vi "Configure Instrument.vi"(8 "error in (no error)":errorcluster, 11 "VNA":refnum<class "VNA.lvclass">) -> (0 "error out":errorcluster, 3 "VNA out":refnum<class "VNA.lvclass">)   [LabVIEW 2019, in "VNA.lvclass"]
uses:
  VNA.lvclass
  <userlib>/LevyLab/Instrument Framework/Instrument Types/VNA/Instrument.VNA.lvclass
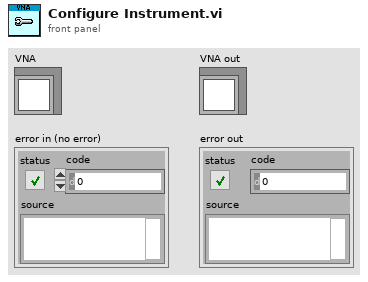
[diagram p1: front panel]
types:
  T1 = typedef "VNA.lvclass/VNA.Configuration--Cluster.ctl" = cluster{"Power":dbl, "Measurement":dbl, "Format":dbl, "Start Freq":dbl, "Stop Freq":dbl, "Num Points":dbl, "Avg Factor":dbl, "Avg?":bool, "Path":path}
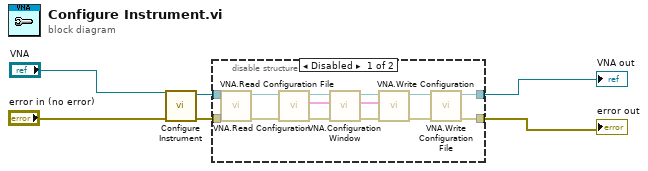
[diagram p0: block diagram]
diagram:
  n1 = call-parent "Configure Instrument.vi"("error in (no error)"="error in (no error)", "Instrument in"="VNA") -> ("error out"=w1:errorcluster, "Instrument out"=w3:refnum<class "VNA.lvclass">)  [unwired: 8 in]
  n2 = disable-structure shown="Disabled" {
    disable-tunnel: [w20 w21] -> w5
    disable-tunnel: [w19 w22] -> w4
    disable-tunnel: w3 -> [w18 w22]
    disable-tunnel: w1 -> [w17 w21]
    frame Disabled {
      n3 = call "VNA.Read Configuration File.vi"("error in (no error)"=w17, "VNA"=w18) -> ("error out"=w16:errorcluster, "VNA out"=w15:refnum<class "VNA.lvclass">)  [unwired: 8 in]
      n4 = call "VNA.Read Configuration.vi"("error in (no error)"=w16, "VNA"=w15) -> ("error out"=w13:errorcluster, "Configuration"=w8:T1, "VNA out"=w14:refnum<class "VNA.lvclass">)  [unwired: 7 in]
      n5 = call "VNA.Configuration Window.vi"("error in (no error)"=w13, "Ex Configuration"=w8, "VNA"=w14) -> ("error out"=w12:errorcluster, "output cluster"=w7:T1, "VNA out"=w11:refnum<class "VNA.lvclass">)  [unwired: 6 in]
      n6 = call "VNA.Write Configuration.vi"("error in (no error)"=w12, "Configuration"=w7, "VNA"=w11) -> ("error out"=w9:errorcluster, "VNA out"=w10:refnum<class "VNA.lvclass">)  [unwired: 7 in]
      n7 = call "VNA.Write Configuration File.vi"("error in (no error)"=w9, "VNA"=w10) -> ("error out"=w20:errorcluster, "VNA out"=w19:refnum<class "VNA.lvclass">)  [unwired: 8 in]
    }
    frame Enabled {
    }
  }
  "error out" <- w5
  "VNA out" <- w4
